vi "Autonomous Independent.vi"   [LabVIEW 2017] (continued)
                tunnel: w5039 -> [w5058]
                tunnel: w5038 -> [w5059]
                tunnel: [w5067] -> w5030
                tunnel: [w5066] -> w5031
                tunnel: [w5064] -> w5032
                tunnel: [w5065] -> w5033
                tunnel: w5037 -> [w5071]
                tunnel: w5036 -> [w5068]
                tunnel: w5035 -> [w5069]
                tunnel: w5034 -> [w5070]
                tunnel: [w5079] -> w5029
                tunnel: w5033 -> [w5075]
                tunnel: w5032 -> [w5076]
                tunnel: w5031 -> [w5078]
                tunnel: w5030 -> [w5080]
                tunnel: [w5077] -> w5028
                tunnel: [w5076] -> w5027
                tunnel: [w5075] -> w5026
                tunnel: w5029 -> [w5090]
                tunnel: [w5090] -> w5025
                tunnel: w5028 -> [w5089]
                tunnel: [w5089] -> w5024
                tunnel: [w5088] -> w5023
                tunnel: [w5087] -> w5022
                tunnel: w5027 -> [w5085]
                tunnel: w5026 -> [w5084]
                tunnel: w5025 -> [w5096]
                tunnel: [w5094] -> w5021
                tunnel: w5024 -> [w5095]
                tunnel: [w5093] -> w5020
                tunnel: w5023 -> [w5098]
                tunnel: w5022 -> [w5097]
                tunnel: [w5092] -> w5019
                tunnel: [w5091] -> w5018
                tunnel: w5021 -> [w5105]
                tunnel: [w5104] -> w5017
                tunnel: [w5103] -> w5016
                tunnel: w5020 -> [w5103]
                tunnel: [w5102] -> w5015
                tunnel: w5019 -> [w5102]
                tunnel: [w5101] -> w5014
                tunnel: w5018 -> [w5101]
                tunnel: [w5116] -> w5013
                tunnel: w5017 -> [w5116]
                tunnel: [w5115] -> w5012
                tunnel: w5016 -> [w5115]
                tunnel: [w5114] -> w5011
                tunnel: w5015 -> [w5114]
                tunnel: [w5113] -> w5010
                tunnel: w5014 -> [w5113]
                tunnel: w5013 -> [w5121]
                tunnel: w5012 -> [w5122]
                tunnel: [w5122] -> w5009
                tunnel: [w5121] -> w5008
                tunnel: [w5120] -> w5007
                tunnel: w5011 -> [w5120]
                tunnel: [w5119] -> w5006
                tunnel: w5010 -> [w5119]
                tunnel: [w5135] -> w5005
                tunnel: w5009 -> [w5137]
                tunnel: w5008 -> [w5136]
                tunnel: w5007 -> [w5132]
                tunnel: w5006 -> [w5131]
                tunnel: [w5130] -> w5004
                tunnel: [w5129] -> w5003
                tunnel: [w5128] -> w5002
                tunnel: w4997 -> [_]
                tunnel: w5005 -> [_]
                tunnel: w5004 -> [_]
                tunnel: w5003 -> [_]
                tunnel: w5002 -> [_]
                frame #0 {
                  n1471 = call "PID Distance.vi"("Distance"=20.0, "Angle"=2.0, "RightEncoder"=w5042, "LeftEncoder"=w5043, "GyroDevRef"=w5044, "RobotDriveDevRef"=w5045) -> ("RightEncoder 2"=w5046:T11, "LeftEncoder 2"=w5047:T11, "GyroDevRef 2"=w5048:T8, "RobotDriveDevRef 2"=w5049:T1)  [unwired: 2 in]
                }
                frame #1 {
                  n1472 = call "PID Distance.vi"("Distance"=100.0, "Angle"=2.0, "RightEncoder"=w5057, "LeftEncoder"=w5058, "GyroDevRef"=w5059, "RobotDriveDevRef"=w5060) -> ("RightEncoder 2"=w5053:T11, "LeftEncoder 2"=w5054:T11, "GyroDevRef 2"=w5055:T8, "RobotDriveDevRef 2"=w5056:T1)  [unwired: 2 in]
                  n1473 = global write "Robot Global Data.vi" "Raise_Mast"(TRUE ("Current State")) -> ()
                }
                frame #2 {
                  n1474 = global write "Robot Global Data.vi" "Lift_Position"(2.0) -> ()
                  n1475 = call "PID Distance.vi"("Distance"=300.0, "Angle"=2.0, "RightEncoder"=w5068, "LeftEncoder"=w5069, "GyroDevRef"=w5070, "RobotDriveDevRef"=w5071) -> ("RightEncoder 2"=w5064:T11, "LeftEncoder 2"=w5065:T11, "GyroDevRef 2"=w5066:T8, "RobotDriveDevRef 2"=w5067:T1)  [unwired: 2 in]
                  n1476 = global write "Robot Global Data.vi" "Raise_Mast"(TRUE ("Current State")) -> ()
                }
                frame #3 {
                  n1477 = global write "Robot Global Data.vi" "Lift_Position"(3.0) -> ()
                  n1478 = call "PID turning.vi"("Angle"=-90.0, "GyroDevRef"=w5078, "RobotDriveDevRef"=w5080) -> ("GyroDevRef 2"=w5077:T8, "RobotDriveDevRef 2"=w5079:T1)  [unwired: 7 in]
                  n1479 = global write "Robot Global Data.vi" "Raise_Mast"(TRUE ("Current State")) -> ()
                }
                frame #4 {
                  n1480 = call <vilib>:"WPI_EncoderReset.vi"("EncoderDevRef"=w5084) -> ("EncoderDevRef"=w5087:T11)  [unwired: 9 in, 1 out]
                  n1481 = Wait (ms)(milliseconds to wait=u32 10) -> ()  [unwired: 1 out]
                  n1482 = call <vilib>:"WPI_EncoderReset.vi"("EncoderDevRef"=w5085) -> ("EncoderDevRef"=w5088:T11)  [unwired: 9 in, 1 out]
                }
                frame #5 {
                  n1483 = call "PID Distance.vi"("Distance"=25.0, "Angle"=-90.0, "RightEncoder"=w5098, "LeftEncoder"=w5097, "GyroDevRef"=w5095, "RobotDriveDevRef"=w5096) -> ("RightEncoder 2"=w5091:T11, "LeftEncoder 2"=w5092:T11, "GyroDevRef 2"=w5093:T8, "RobotDriveDevRef 2"=w5094:T1)  [unwired: 2 in]
                }
                frame #6 {
                  w5106 = 0.0 ("Left axis value")
                  n1484 = global read "Robot Global Data.vi" "Axes"() -> (w5109:dbl[])
                  n1485 = Wait (ms)(milliseconds to wait=u32 500) -> ()  [unwired: 1 out]
                  n1486 = Array To Cluster(array=w5109) -> (cluster=w5108:T15)
                  n1487 = Bundle By Name(cluster=w5108, "Axes[1]"=0.25) -> (w5111:T15)
                  n1488 = Cluster To Array(cluster=w5111) -> (array=w5110:dbl[])
                  n1489 = call <vilib>:"WPI_RobotDriveTankDrive.vi"("Right axis value"=w5106, "Left axis value"=w5106, "RobotDriveDevRef"=w5105) -> ("RobotDriveDevRef"=w5104:T1)  [unwired: 6 in, 2 out]
                  n1490 = global write "Robot Global Data.vi" "Axes"(w5110) -> ()
                }
                frame #7 {
                  n1491 = global write "Robot Global Data.vi" "Current State"(FALSE ("Current State")) -> ()
                  n1492 = Wait (ms)(milliseconds to wait=u32 400) -> ()  [unwired: 1 out]
                }
                frame #8 {
                  n1493 = global read "Robot Global Data.vi" "Axes"() -> (w5124:dbl[])
                  n1494 = Array To Cluster(array=w5124) -> (cluster=w5123:T15)
                  n1495 = Bundle By Name(cluster=w5123, "Axes[1]"=-1.0) -> (w5126:T15)
                  n1496 = Cluster To Array(cluster=w5126) -> (array=w5125:dbl[])
                  n1497 = global write "Robot Global Data.vi" "Axes"(w5125) -> ()
                }
                frame #9 {
                  n1498 = call "PID Distance.vi"("Distance"=0.0, "Angle"=-90.0, "RightEncoder"=w5131, "LeftEncoder"=w5132, "GyroDevRef"=w5137, "RobotDriveDevRef"=w5136) -> ("RightEncoder 2"=w5128:T11, "LeftEncoder 2"=w5129:T11, "GyroDevRef 2"=w5130:T8, "RobotDriveDevRef 2"=w5135:T1)  [unwired: 2 in]
                }
                frame #10 {
                  n1499 = global write "Robot Global Data.vi" "Lift_Position"(1.0) -> ()
                }
              }
            }
            frame Default {
              n1500 = flat-sequence {
                tunnel: w5142 -> [w5148]
                tunnel: w5141 -> [w5147]
                tunnel: w5140 -> [w5145]
                tunnel: [w5146] -> w5143
                tunnel: w5139 -> [w5144]
                tunnel: w5143 -> [w5151]
                frame #0 {
                  n1501 = call "PID Distance.vi"("Distance"=90.0, "Angle"=0.0, "RightEncoder"=w5144, "LeftEncoder"=w5145, "GyroDevRef"=w5147, "RobotDriveDevRef"=w5148) -> ("RobotDriveDevRef 2"=w5146:T1)  [unwired: 2 in, 3 out]
                }
                frame #1 {
                  w5152 = 0.0
                  n1502 = call <vilib>:"WPI_RobotDriveTankDrive.vi"("Right axis value"=w5152, "Left axis value"=w5152, "RobotDriveDevRef"=w5151) -> ()  [unwired: 6 in, 3 out]
                }
              }
            }
          }
        }
      }
    }
    frame "Right Scale 2" {
      n1503 = flat-sequence {
        tunnel: w5158 -> [w5188]
        tunnel: w5155 -> [w5186]
        tunnel: w5156 -> [w5185]
        tunnel: w5157 -> [w5184]
        tunnel: [w5183] -> w5163
        tunnel: [w5182] -> w5162
        tunnel: [w5181] -> w5161
        tunnel: [w5180] -> w5160
        tunnel: w5159 -> [w5173]
        tunnel: w5154 -> [w5190]
        tunnel: w5163 -> [w5194]
        tunnel: w5162 -> [w5193]
        tunnel: w5161 -> [w5192]
        tunnel: w5160 -> [w5191]
        tunnel: w5153 -> [w5189]
        frame #0 {
          w5187 = 0.0 ("Left axis value")
          n1504 = global read "Robot Global Data.vi" "Axes"() -> (w5166:dbl[])
          n1505 = Multiply(x=w5173, y=1000.0) -> (x*y=w5174:dbl)
          n1506 = global write "Robot Global Data.vi" "Lift_Position"(0.0) -> ()
          n1507 = global write "Robot Global Data.vi" "Current State"(TRUE ("Current State")) -> ()
          n1508 = global write "Robot Global Data.vi" "Raise_Mast"(FALSE ("Current State")) -> ()
          n1509 = Wait (ms)(milliseconds to wait=u32 100) -> ()  [unwired: 1 out]
          n1510 = Array To Cluster(array=w5166) -> (cluster=w5165:T15)
          n1511 = Bundle By Name(cluster=w5165, "Axes[1]"=-1.0) -> (w5168:T15)
          n1512 = Greater?(x=w5174, y=11000.0) -> (0:w5176:bool)
          n1513 = Equal?(x=w5174, y=0.0) -> (x = y?=w5177:bool)
          n1514 = Or(x=w5176, y=w5177) -> ()  [unwired: 1 out]
          n1515 = Cluster To Array(cluster=w5168) -> (array=w5167:dbl[])
          n1516 = call <vilib>:"WPI_GyroReset.vi"("GyroDevRef"=w5184) -> ("GyroDevRef"=w5180:T8)  [unwired: 9 in, 1 out]
          n1517 = call <vilib>:"WPI_EncoderReset.vi"("EncoderDevRef"=w5186) -> ("EncoderDevRef"=w5182:T11)  [unwired: 9 in, 1 out]
          n1518 = global write "Robot Global Data.vi" "Axes"(w5167) -> ()
          n1519 = call <vilib>:"WPI_EncoderReset.vi"("EncoderDevRef"=w5185) -> ("EncoderDevRef"=w5181:T11)  [unwired: 9 in, 1 out]
          n1520 = call <vilib>:"WPI_RobotDriveTankDrive.vi"("Right axis value"=w5187, "Left axis value"=w5187, "RobotDriveDevRef"=w5188) -> ("RobotDriveDevRef"=w5183:T1)  [unwired: 6 in, 2 out]
        }
        frame #1 {
          n1521 = case shown="\"L\"" w5190 {
            tunnel: w5194 -> [w5196 w5543 w5871]
            tunnel: w5193 -> [w5199 w5540 w5873]
            tunnel: w5192 -> [w5198 w5541 w5872]
            tunnel: w5191 -> [w5197 w5542 w5870]
            tunnel: w5189 -> [w5195 w5539 _]
            frame "L" {
              n1522 = flat-sequence {
                tunnel: w5199 -> [w5261]
                tunnel: w5198 -> [w5262]
                tunnel: w5197 -> [w5263]
                tunnel: w5196 -> [w5264]
                tunnel: [w5257] -> w5255
                tunnel: [w5258] -> w5254
                tunnel: [w5259] -> w5253
                tunnel: [w5260] -> w5252
                tunnel: [w5274] -> w5251
                tunnel: [w5273] -> w5250
                tunnel: [w5271] -> w5249
                tunnel: [w5272] -> w5248
                tunnel: w5255 -> [w5270]
                tunnel: w5254 -> [w5269]
                tunnel: w5253 -> [w5268]
                tunnel: w5252 -> [w5267]
                tunnel: w5251 -> [w5280]
                tunnel: w5250 -> [w5281]
                tunnel: [w5284] -> w5247
                tunnel: w5249 -> [w5284]
                tunnel: [w5283] -> w5246
                tunnel: w5248 -> [w5283]
                tunnel: [w5278] -> w5245
                tunnel: [w5279] -> w5244
                tunnel: w5247 -> [w5291]
                tunnel: w5246 -> [w5290]
                tunnel: [w5289] -> w5243
                tunnel: [w5288] -> w5242
                tunnel: [w5287] -> w5241
                tunnel: w5245 -> [w5287]
                tunnel: [w5285] -> w5240
                tunnel: w5244 -> [w5285]
                tunnel: w5243 -> [w5296]
                tunnel: w5242 -> [w5297]
                tunnel: w5241 -> [w5298]
                tunnel: [w5294] -> w5239
                tunnel: [w5295] -> w5238
                tunnel: w5240 -> [w5299]
                tunnel: [w5292] -> w5237
                tunnel: [w5293] -> w5236
                tunnel: w5239 -> [w5311]
                tunnel: w5238 -> [w5310]
                tunnel: [w5309] -> w5235
                tunnel: [w5308] -> w5234
                tunnel: [w5314] -> w5233
                tunnel: w5237 -> [w5314]
                tunnel: [w5313] -> w5232
                tunnel: w5236 -> [w5313]
                tunnel: w5235 -> [w5320]
                tunnel: [w5320] -> w5231
                tunnel: [w5319] -> w5230
                tunnel: [w5318] -> w5229
                tunnel: [w5317] -> w5228
                tunnel: w5234 -> [w5317]
                tunnel: w5233 -> [w5316]
                tunnel: w5232 -> [w5315]
                tunnel: w5231 -> [w5328]
                tunnel: [w5325] -> w5227
                tunnel: w5230 -> [w5327]
                tunnel: w5229 -> [w5326]
                tunnel: w5228 -> [w5329]
                tunnel: [w5324] -> w5226
                tunnel: [w5323] -> w5225
                tunnel: [w5322] -> w5224
                tunnel: w5227 -> [w5336]
                tunnel: [w5335] -> w5223
                tunnel: w5226 -> [w5333]
                tunnel: [w5332] -> w5222
                tunnel: w5225 -> [w5338]
                tunnel: [w5338] -> w5221
                tunnel: w5224 -> [w5337]
                tunnel: [w5337] -> w5220
                tunnel: w5223 -> [w5349]
                tunnel: [w5343] -> w5219
                tunnel: [w5342] -> w5218
                tunnel: w5222 -> [w5342]
                tunnel: [w5341] -> w5217
                tunnel: w5221 -> [w5341]
                tunnel: [w5340] -> w5216
                tunnel: w5220 -> [w5340]
                tunnel: w5219 -> [w5356]
                tunnel: [w5356] -> w5215
                tunnel: w5218 -> [w5355]
                tunnel: [w5355] -> w5214
                tunnel: w5217 -> [w5354]
                tunnel: [w5354] -> w5213
                tunnel: w5216 -> [w5353]
                tunnel: [w5353] -> w5212
                tunnel: w5215 -> [w5360]
                tunnel: [w5358] -> w5211
                tunnel: w5214 -> [w5359]
                tunnel: [w5357] -> w5210
                tunnel: w5213 -> [w5363]
                tunnel: [w5363] -> w5209
                tunnel: w5212 -> [w5362]
                tunnel: [w5362] -> w5208
                tunnel: w5211 -> [w5376]
                tunnel: w5210 -> [w5375]
                tunnel: w5209 -> [w5374]
                tunnel: w5208 -> [w5373]
                tunnel: [w5367] -> w5207
                tunnel: [w5366] -> w5206
                tunnel: [w5365] -> w5205
                tunnel: [w5364] -> w5204
                tunnel: w5207 -> [w5383]
                tunnel: [w5383] -> w5203
                tunnel: w5206 -> [w5382]
                tunnel: [w5382] -> w5202
                tunnel: w5205 -> [w5381]
                tunnel: [w5381] -> w5201
                tunnel: w5204 -> [w5380]
                tunnel: [w5380] -> w5200
                tunnel: w5203 -> [w5388]
                tunnel: w5202 -> [w5387]
                tunnel: w5201 -> [w5385]
                tunnel: w5200 -> [w5386]
                tunnel: w5195 -> [w5384]
                frame #0 {
                  n1523 = global write "Robot Global Data.vi" "Raise_Mast"(FALSE ("Current State")) -> ()
                  n1524 = call "PID Distance.vi"("Distance"=20.0, "Angle"=0.0, "RightEncoder"=w5261, "LeftEncoder"=w5262, "GyroDevRef"=w5263, "RobotDriveDevRef"=w5264) -> ("RightEncoder 2"=w5260:T11, "LeftEncoder 2"=w5259:T11, "GyroDevRef 2"=w5258:T8, "RobotDriveDevRef 2"=w5257:T1)  [unwired: 2 in]
                }
                frame #1 {
                  n1525 = global write "Robot Global Data.vi" "Raise_Mast"(TRUE ("Current State")) -> ()
                  n1526 = call "PID Distance.vi"("Distance"=225.0, "Angle"=0.0, "RightEncoder"=w5267, "LeftEncoder"=w5268, "GyroDevRef"=w5269, "RobotDriveDevRef"=w5270) -> ("RightEncoder 2"=w5271:T11, "LeftEncoder 2"=w5272:T11, "GyroDevRef 2"=w5273:T8, "RobotDriveDevRef 2"=w5274:T1)  [unwired: 2 in]
                }
                frame #2 {
                  n1527 = call "PID turning.vi"("Angle"=-90.0, "GyroDevRef"=w5281, "RobotDriveDevRef"=w5280) -> ("GyroDevRef 2"=w5278:T8, "RobotDriveDevRef 2"=w5279:T1)  [unwired: 7 in]
                }
                frame #3 {
                  n1528 = call <vilib>:"WPI_EncoderReset.vi"("EncoderDevRef"=w5290) -> ("EncoderDevRef"=w5288:T11)  [unwired: 9 in, 1 out]
                  n1529 = Wait (ms)(milliseconds to wait=u32 10) -> ()  [unwired: 1 out]
                  n1530 = call <vilib>:"WPI_EncoderReset.vi"("EncoderDevRef"=w5291) -> ("EncoderDevRef"=w5289:T11)  [unwired: 9 in, 1 out]
                }
                frame #4 {
                  n1531 = global read "Robot Global Data.vi" "Axes"() -> (w5303:dbl[])
                  n1532 = global write "Robot Global Data.vi" "Lift_Position"(2.0) -> ()
                  n1533 = call "PID Distance.vi"("Distance"=199.0, "Angle"=-90.0, "RightEncoder"=w5296, "LeftEncoder"=w5297, "GyroDevRef"=w5298, "RobotDriveDevRef"=w5299) -> ("RightEncoder 2"=w5293:T11, "LeftEncoder 2"=w5292:T11, "GyroDevRef 2"=w5295:T8, "RobotDriveDevRef 2"=w5294:T1)  [unwired: 2 in]
                  n1534 = Array To Cluster(array=w5303) -> (cluster=w5302:T15)
                  n1535 = Bundle By Name(cluster=w5302, "Axes[1]"=-1.0) -> (w5301:T15)
                  n1536 = Cluster To Array(cluster=w5301) -> (array=w5300:dbl[])
                  n1537 = global write "Robot Global Data.vi" "Axes"(w5300) -> ()
                }
                frame #5 {
                  n1538 = call "PID turning.vi"("Angle"=0.0, "GyroDevRef"=w5310, "RobotDriveDevRef"=w5311) -> ("GyroDevRef 2"=w5308:T8, "RobotDriveDevRef 2"=w5309:T1)  [unwired: 7 in]
                }
                frame #6 {
                  n1539 = call <vilib>:"WPI_EncoderReset.vi"("EncoderDevRef"=w5316) -> ("EncoderDevRef"=w5319:T11)  [unwired: 9 in, 1 out]
                  n1540 = call <vilib>:"WPI_EncoderReset.vi"("EncoderDevRef"=w5315) -> ("EncoderDevRef"=w5318:T11)  [unwired: 9 in, 1 out]
                }
                frame #7 {
                  n1541 = call "PID Distance.vi"("Distance"=38.0, "Angle"=0.0, "RightEncoder"=w5326, "LeftEncoder"=w5327, "GyroDevRef"=w5329, "RobotDriveDevRef"=w5328) -> ("RightEncoder 2"=w5322:T11, "LeftEncoder 2"=w5323:T11, "GyroDevRef 2"=w5324:T8, "RobotDriveDevRef 2"=w5325:T1)  [unwired: 2 in]
                  n1542 = global write "Robot Global Data.vi" "Lift_Position"(3.0) -> ()
                }
                frame #8 {
                  n1543 = call "PID turning.vi"("Angle"=20.0, "GyroDevRef"=w5333, "RobotDriveDevRef"=w5336) -> ("GyroDevRef 2"=w5332:T8, "RobotDriveDevRef 2"=w5335:T1)  [unwired: 7 in]
                }
                frame #9 {
                  w5350 = 0.0 ("Left axis value")
                  n1544 = global read "Robot Global Data.vi" "Axes"() -> (w5345:dbl[])
                  n1545 = Wait (ms)(milliseconds to wait=u32 300) -> ()  [unwired: 1 out]
                  n1546 = Array To Cluster(array=w5345) -> (cluster=w5344:T15)
                  n1547 = Bundle By Name(cluster=w5344, "Axes[1]"=0.25) -> (w5347:T15)
                  n1548 = Cluster To Array(cluster=w5347) -> (array=w5346:dbl[])
                  n1549 = call <vilib>:"WPI_RobotDriveTankDrive.vi"("Right axis value"=w5350, "Left axis value"=w5350, "RobotDriveDevRef"=w5349) -> ("RobotDriveDevRef"=w5343:T1)  [unwired: 6 in, 2 out]
                  n1550 = global write "Robot Global Data.vi" "Axes"(w5346) -> ()
                }
                frame #10 {
                  n1551 = global write "Robot Global Data.vi" "Current State"(FALSE ("Current State")) -> ()
                  n1552 = Wait (ms)(milliseconds to wait=u32 400) -> ()  [unwired: 1 out]
                }
                frame #11 {
                  n1553 = call "PID turning.vi"("Angle"=0.0, "GyroDevRef"=w5359, "RobotDriveDevRef"=w5360) -> ("GyroDevRef 2"=w5357:T8, "RobotDriveDevRef 2"=w5358:T1)  [unwired: 7 in]
                }
                frame #12 {
                  n1554 = global read "Robot Global Data.vi" "Axes"() -> (w5372:dbl[])
                  n1555 = Array To Cluster(array=w5372) -> (cluster=w5371:T15)
                  n1556 = call "PID Distance.vi"("Distance"=0.0, "Angle"=0.0, "RightEncoder"=w5373, "LeftEncoder"=w5374, "GyroDevRef"=w5375, "RobotDriveDevRef"=w5376) -> ("RightEncoder 2"=w5364:T11, "LeftEncoder 2"=w5365:T11, "GyroDevRef 2"=w5366:T8, "RobotDriveDevRef 2"=w5367:T1)  [unwired: 2 in]
                  n1557 = Bundle By Name(cluster=w5371, "Axes[1]"=-1.0) -> (w5370:T15)
                  n1558 = Cluster To Array(cluster=w5370) -> (array=w5369:dbl[])
                  n1559 = global write "Robot Global Data.vi" "Axes"(w5369) -> ()
                }
                frame #13 {
                  n1560 = global write "Robot Global Data.vi" "Lift_Position"(1.0) -> ()
                }
                frame #14 {
                  n1561 = case shown="\"L\"" w5384 {
                    tunnel: w5388 -> [w5392 w5463 _]
                    tunnel: w5387 -> [w5391 w5462 _]
                    tunnel: w5386 -> [w5390 w5459 _]
                    tunnel: w5385 -> [w5389 w5458 _]
                    frame "R" {
                      n1562 = flat-sequence {
                        tunnel: w5392 -> [w5401]
                        tunnel: w5391 -> [w5400]
                        tunnel: [w5403] -> w5398
                        tunnel: [w5402] -> w5397
                        tunnel: w5398 -> [w5410]
                        tunnel: w5397 -> [w5409]
                        tunnel: [w5410] -> w5393
                        tunnel: [w5409] -> w5394
                        tunnel: [w5407] -> w5395
                        tunnel: [w5406] -> w5396
                        tunnel: w5390 -> [w5405]
                        tunnel: w5389 -> [w5404]
                        tunnel: w5396 -> [w5412]
                        tunnel: w5395 -> [w5413]
                        tunnel: w5394 -> [w5414]
                        tunnel: w5393 -> [w5415]
                        frame #0 {
                          n1563 = call "PID turning.vi"("Angle"=170.0, "GyroDevRef"=w5400, "RobotDriveDevRef"=w5401) -> ("GyroDevRef 2"=w5402:T8, "RobotDriveDevRef 2"=w5403:T1)  [unwired: 7 in]
                        }
                        frame #1 {
                          n1564 = call <vilib>:"WPI_EncoderReset.vi"("EncoderDevRef"=w5405) -> ("EncoderDevRef"=w5406:T11)  [unwired: 9 in, 1 out]
                          n1565 = Wait (ms)(milliseconds to wait=u32 10) -> ()  [unwired: 1 out]
                          n1566 = call <vilib>:"WPI_EncoderReset.vi"("EncoderDevRef"=w5404) -> ("EncoderDevRef"=w5407:T11)  [unwired: 9 in, 1 out]
                        }
                        frame #2 {
                          n1567 = global read "Robot Global Data.vi" "Axes"() -> (w5421:dbl[])
                          n1568 = Wait (ms)(milliseconds to wait=u32 400) -> ()  [unwired: 1 out]
                          n1569 = Array To Cluster(array=w5421) -> (cluster=w5422:T15)
                          n1570 = Bundle By Name(cluster=w5422, "Axes[1]"=1.0) -> (w5423:T15)
                          n1571 = global read "Robot Global Data.vi" "PIXY Output"() -> (w5411:T16)
                          n1572 = Unbundle By Name(w5411) -> ("SIGNATURE NUMBER"=w5418:u16)
                          n1573 = global read "Robot Global Data.vi" "Cube Signature"() -> (w5416:dbl)
                          n1574 = Equal?(x=w5418, y=w5416) -> (x = y?=w5417:bool)
                          n1575 = Cluster To Array(cluster=w5423) -> (array=w5424:dbl[])
                          n1576 = global write "Robot Global Data.vi" "Axes"(w5424) -> ()
                          n1577 = case shown="False" w5417 {
                            tunnel: [w5426 w5439] -> _
                            tunnel: [w5425 w5438] -> _
                            tunnel: [w5428 w5437] -> _
                            tunnel: [w5429 w5436] -> _
                            tunnel: w5415 -> [w5427 w5433]
                            tunnel: w5414 -> [w5428 w5432]
                            tunnel: w5413 -> [w5425 w5431]
                            tunnel: w5412 -> [w5426 w5430]
                            frame True {
                              n1578 = call "PID vision.vi"("RobotDriveDevRef in"=w5427) -> ("RobotDriveDevRef out"=w5429:T1)  [unwired: 9 in, 1 out]
                            }
                            frame False {
                              n1579 = call "PID Distance.vi"("Distance"=45.0, "Angle"=170.0, "RightEncoder"=w5430, "LeftEncoder"=w5431, "GyroDevRef"=w5432, "RobotDriveDevRef"=w5433) -> ("RightEncoder 2"=w5439:T11, "LeftEncoder 2"=w5438:T11, "GyroDevRef 2"=w5437:T8, "RobotDriveDevRef 2"=w5436:T1)  [unwired: 2 in]
                            }
                          }
                        }
                        frame #3 {
                          n1580 = global write "Robot Global Data.vi" "Current State"(TRUE ("Current State")) -> ()
                          n1581 = Wait (ms)(milliseconds to wait=u32 300) -> ()  [unwired: 1 out]
                        }
                      }
                    }
                    frame "L" {
                      n1582 = flat-sequence {
                        tunnel: w5463 -> [w5466]
                        tunnel: w5462 -> [w5465]
                        tunnel: [w5468] -> w5461
                        tunnel: [w5467] -> w5460
                        tunnel: w5461 -> [w5475]
                        tunnel: w5460 -> [w5474]
                        tunnel: w5459 -> [w5472]
                        tunnel: w5458 -> [w5471]
                        tunnel: [w5475] -> w5457
                        tunnel: [w5474] -> w5456
                        tunnel: [w5470] -> w5455
                        tunnel: [w5469] -> w5454
                        tunnel: [w5493] -> w5453
                        tunnel: [w5492] -> w5452
                        tunnel: [w5491] -> w5451
                        tunnel: [w5490] -> w5450
                        tunnel: w5454 -> [w5482]
                        tunnel: w5455 -> [w5483]
                        tunnel: w5456 -> [w5481]
                        tunnel: w5457 -> [w5480]
                        tunnel: w5453 -> [w5514]
                        tunnel: w5452 -> [w5513]
                        tunnel: w5451 -> [w5512]
                        tunnel: w5450 -> [w5511]
                        tunnel: [w5514] -> w5449
                        tunnel: [w5513] -> w5447
                        tunnel: [w5512] -> w5445
                        tunnel: [w5511] -> w5443
                        tunnel: w5449 -> [w5525]
                        tunnel: [w5525] -> w5448
                        tunnel: w5447 -> [w5524]
                        tunnel: [w5524] -> w5446
                        tunnel: w5445 -> [w5523]
                        tunnel: [w5523] -> w5444
                        tunnel: w5443 -> [w5522]
                        tunnel: [w5522] -> w5442
                        tunnel: w5448 -> [w5526]
                        tunnel: w5446 -> [w5529]
                        tunnel: w5444 -> [w5528]
                        tunnel: w5442 -> [w5527]
                        frame #0 {
                          n1583 = call "PID turning.vi"("Angle"=170.0, "GyroDevRef"=w5465, "RobotDriveDevRef"=w5466) -> ("GyroDevRef 2"=w5467:T8, "RobotDriveDevRef 2"=w5468:T1)  [unwired: 7 in]
                        }
                        frame #1 {
                          n1584 = call <vilib>:"WPI_EncoderReset.vi"("EncoderDevRef"=w5471) -> ("EncoderDevRef"=w5469:T11)  [unwired: 9 in, 1 out]
                          n1585 = Wait (ms)(milliseconds to wait=u32 10) -> ()  [unwired: 1 out]
                          n1586 = call <vilib>:"WPI_EncoderReset.vi"("EncoderDevRef"=w5472) -> ("EncoderDevRef"=w5470:T11)  [unwired: 9 in, 1 out]
                        }
                        frame #2 {
                          n1587 = global read "Robot Global Data.vi" "Axes"() -> (w5486:dbl[])
                          n1588 = Wait (ms)(milliseconds to wait=u32 400) -> ()  [unwired: 1 out]
                          n1589 = Array To Cluster(array=w5486) -> (cluster=w5487:T15)
                          n1590 = Bundle By Name(cluster=w5487, "Axes[1]"=1.0) -> (w5488:T15)
                          n1591 = global read "Robot Global Data.vi" "PIXY Output"() -> (w5476:T16)
                          n1592 = Unbundle By Name(w5476) -> ("SIGNATURE NUMBER"=w5479:u16)
                          n1593 = global read "Robot Global Data.vi" "Cube Signature"() -> (w5477:dbl)
                          n1594 = Equal?(x=w5479, y=w5477) -> (x = y?=w5478:bool)
                          n1595 = Cluster To Array(cluster=w5488) -> (array=w5489:dbl[])
                          n1596 = global write "Robot Global Data.vi" "Axes"(w5489) -> ()
                          n1597 = case shown="True" w5478 {
                            tunnel: [w5495 w5508] -> w5493
                            tunnel: [w5494 w5507] -> w5492
                            tunnel: [w5496 w5506] -> w5491
                            tunnel: [w5497 w5505] -> w5490
                            tunnel: w5483 -> [w5494 w5502]
                            tunnel: w5482 -> [w5495 w5501]
                            tunnel: w5481 -> [w5496 w5500]
                            tunnel: w5480 -> [w5498 w5499]
                            frame True {
                              (unwired) 10.0 ("Distance")
                              n1598 = call "PID vision.vi"("RobotDriveDevRef in"=w5498) -> ("RobotDriveDevRef out"=w5497:T1)  [unwired: 9 in, 1 out]
                            }
                            frame False {
                              n1599 = call "PID Distance.vi"("Distance"=45.0, "Angle"=170.0, "RightEncoder"=w5502, "LeftEncoder"=w5501, "GyroDevRef"=w5500, "RobotDriveDevRef"=w5499) -> ("RightEncoder 2"=w5508:T11, "LeftEncoder 2"=w5507:T11, "GyroDevRef 2"=w5506:T8, "RobotDriveDevRef 2"=w5505:T1)  [unwired: 2 in]
                            }
                          }
                        }
                        frame #3 {
                          n1600 = global write "Robot Global Data.vi" "Current State"(TRUE ("Current State")) -> ()
                          n1601 = Wait (ms)(milliseconds to wait=u32 500) -> ()  [unwired: 1 out]
                        }
                        frame #4 {
                          n1602 = global read "Robot Global Data.vi" "Axes"() -> (w5520:dbl[])
                          n1603 = global write "Robot Global Data.vi" "Lift_Position"(2.0) -> ()
                          n1604 = Wait (ms)(milliseconds to wait=u32 250) -> ()  [unwired: 1 out]
                          n1605 = Array To Cluster(array=w5520) -> (cluster=w5519:T15)
                          n1606 = Bundle By Name(cluster=w5519, "Axes[1]"=-1.0) -> (w5517:T15)
                          n1607 = Cluster To Array(cluster=w5517) -> (array=w5516:dbl[])
                          n1608 = global write "Robot Global Data.vi" "Axes"(w5516) -> ()
                        }
                        frame #5 {
                          n1609 = call "PID Distance.vi"("Distance"=60.0, "Angle"=170.0, "RightEncoder"=w5526, "LeftEncoder"=w5529, "GyroDevRef"=w5528, "RobotDriveDevRef"=w5527) -> ()  [unwired: 2 in, 4 out]
                        }
                        frame #6 {
                          n1610 = global read "Robot Global Data.vi" "Axes"() -> (w5537:dbl[])
                          n1611 = Wait (ms)(milliseconds to wait=u32 250) -> ()  [unwired: 1 out]
                          n1612 = Array To Cluster(array=w5537) -> (cluster=w5536:T15)
                          n1613 = Bundle By Name(cluster=w5536, "Axes[1]"=1.0) -> (w5534:T15)
                          n1614 = Cluster To Array(cluster=w5534) -> (array=w5533:dbl[])
                          n1615 = global write "Robot Global Data.vi" "Axes"(w5533) -> ()
                        }
                        frame #7 {
                          n1616 = global write "Robot Global Data.vi" "Current State"(FALSE ("Current State")) -> ()
                        }
                      }
                    }
                    frame Default {
                    }
                  }
                }
              }
            }
            frame "R" {
              n1617 = flat-sequence {
                tunnel: [w5607] -> w5599
                tunnel: [w5604] -> w5598
                tunnel: [w5605] -> w5597
                tunnel: [w5606] -> w5596
                tunnel: w5543 -> [w5603]
                tunnel: w5542 -> [w5602]
                tunnel: w5541 -> [w5601]
                tunnel: w5540 -> [w5600]
                tunnel: [w5614] -> w5595
                tunnel: [w5611] -> w5594
                tunnel: [w5612] -> w5593
                tunnel: [w5613] -> w5592
                tunnel: w5599 -> [w5618]
                tunnel: w5598 -> [w5615]
                tunnel: w5597 -> [w5616]
                tunnel: w5596 -> [w5617]
                tunnel: [w5625] -> w5588
                tunnel: [w5624] -> w5589
                tunnel: [w5622] -> w5590
                tunnel: [w5623] -> w5591
                tunnel: w5595 -> [w5629]
                tunnel: w5594 -> [w5626]
                tunnel: w5593 -> [w5627]
                tunnel: w5592 -> [w5628]
                tunnel: [w5637] -> w5587
                tunnel: w5591 -> [w5633]
                tunnel: w5590 -> [w5634]
                tunnel: w5589 -> [w5636]
                tunnel: w5588 -> [w5638]
                tunnel: [w5635] -> w5586
                tunnel: [w5634] -> w5585
                tunnel: [w5633] -> w5584
                tunnel: w5587 -> [w5648]
                tunnel: [w5648] -> w5583
                tunnel: w5586 -> [w5647]
                tunnel: [w5647] -> w5582
                tunnel: [w5646] -> w5581
                tunnel: [w5645] -> w5580
                tunnel: w5585 -> [w5643]
                tunnel: w5584 -> [w5642]
                tunnel: w5583 -> [w5654]
                tunnel: [w5652] -> w5579
                tunnel: w5582 -> [w5653]
                tunnel: [w5651] -> w5578
                tunnel: w5581 -> [w5656]
                tunnel: w5580 -> [w5655]
                tunnel: [w5650] -> w5577
                tunnel: [w5649] -> w5576
                tunnel: w5579 -> [w5663]
                tunnel: [w5662] -> w5575
                tunnel: [w5661] -> w5574
                tunnel: w5578 -> [w5661]
                tunnel: [w5660] -> w5573
                tunnel: w5577 -> [w5660]
                tunnel: [w5659] -> w5572
                tunnel: w5576 -> [w5659]
                tunnel: [w5674] -> w5571
                tunnel: w5575 -> [w5674]
                tunnel: [w5673] -> w5570
                tunnel: w5574 -> [w5673]
                tunnel: [w5672] -> w5569
                tunnel: w5573 -> [w5672]
                tunnel: [w5671] -> w5568
                tunnel: w5572 -> [w5671]
                tunnel: w5571 -> [w5679]
                tunnel: w5570 -> [w5680]
                tunnel: [w5680] -> w5567
                tunnel: [w5679] -> w5566
                tunnel: [w5678] -> w5565
                tunnel: w5569 -> [w5678]
                tunnel: [w5677] -> w5564
                tunnel: w5568 -> [w5677]
                tunnel: [w5693] -> w5563
                tunnel: w5567 -> [w5695]
                tunnel: w5566 -> [w5694]
                tunnel: w5565 -> [w5690]
                tunnel: w5564 -> [w5689]
                tunnel: [w5688] -> w5562
                tunnel: [w5687] -> w5561
                tunnel: [w5686] -> w5560
                tunnel: w5563 -> [w5702]
                tunnel: w5562 -> [w5701]
                tunnel: [w5700] -> w5559
                tunnel: w5561 -> [w5700]
                tunnel: [w5699] -> w5558
                tunnel: w5560 -> [w5699]
                tunnel: [w5698] -> w5557
                tunnel: [w5697] -> w5556
                tunnel: w5559 -> [w5710]
                tunnel: w5558 -> [w5709]
                tunnel: [w5707] -> w5555
                tunnel: w5557 -> [w5707]
                tunnel: [w5706] -> w5554
                tunnel: w5556 -> [w5706]
                tunnel: [w5705] -> w5553
                tunnel: [w5704] -> w5552
                tunnel: w5555 -> [w5723]
                tunnel: w5554 -> [w5722]
                tunnel: w5553 -> [w5721]
                tunnel: w5552 -> [w5720]
                tunnel: [w5719] -> w5551
                tunnel: [w5718] -> w5550
                tunnel: [w5717] -> w5549
                tunnel: [w5716] -> w5548
                tunnel: [w5729] -> w5547
                tunnel: [w5726] -> w5546
                tunnel: [w5728] -> w5545
                tunnel: [w5727] -> w5544
                tunnel: w5548 -> [w5726]
                tunnel: w5549 -> [w5727]
                tunnel: w5550 -> [w5728]
                tunnel: w5551 -> [w5729]
                tunnel: w5547 -> [w5736]
                tunnel: w5546 -> [w5735]
                tunnel: w5545 -> [w5734]
                tunnel: w5544 -> [w5733]
                tunnel: w5539 -> [w5732]
                frame #0 {
                  n1618 = call "PID Distance.vi"("Distance"=20.0, "Angle"=2.0, "RightEncoder"=w5600, "LeftEncoder"=w5601, "GyroDevRef"=w5602, "RobotDriveDevRef"=w5603) -> ("RightEncoder 2"=w5604:T11, "LeftEncoder 2"=w5605:T11, "GyroDevRef 2"=w5606:T8, "RobotDriveDevRef 2"=w5607:T1)  [unwired: 2 in]
                }
                frame #1 {
                  n1619 = call "PID Distance.vi"("Distance"=100.0, "Angle"=2.0, "RightEncoder"=w5615, "LeftEncoder"=w5616, "GyroDevRef"=w5617, "RobotDriveDevRef"=w5618) -> ("RightEncoder 2"=w5611:T11, "LeftEncoder 2"=w5612:T11, "GyroDevRef 2"=w5613:T8, "RobotDriveDevRef 2"=w5614:T1)  [unwired: 2 in]
                  n1620 = global write "Robot Global Data.vi" "Raise_Mast"(TRUE ("Current State")) -> ()
                }
                frame #2 {
                  n1621 = global write "Robot Global Data.vi" "Lift_Position"(2.0) -> ()
                  n1622 = call "PID Distance.vi"("Distance"=300.0, "Angle"=2.0, "RightEncoder"=w5626, "LeftEncoder"=w5627, "GyroDevRef"=w5628, "RobotDriveDevRef"=w5629) -> ("RightEncoder 2"=w5622:T11, "LeftEncoder 2"=w5623:T11, "GyroDevRef 2"=w5624:T8, "RobotDriveDevRef 2"=w5625:T1)  [unwired: 2 in]
                  n1623 = global write "Robot Global Data.vi" "Raise_Mast"(TRUE ("Current State")) -> ()
                }
                frame #3 {
                  n1624 = global write "Robot Global Data.vi" "Lift_Position"(3.0) -> ()
                  n1625 = call "PID turning.vi"("Angle"=-90.0, "GyroDevRef"=w5636, "RobotDriveDevRef"=w5638) -> ("GyroDevRef 2"=w5635:T8, "RobotDriveDevRef 2"=w5637:T1)  [unwired: 7 in]
                  n1626 = global write "Robot Global Data.vi" "Raise_Mast"(TRUE ("Current State")) -> ()
                }
                frame #4 {
                  n1627 = call <vilib>:"WPI_EncoderReset.vi"("EncoderDevRef"=w5642) -> ("EncoderDevRef"=w5645:T11)  [unwired: 9 in, 1 out]
                  n1628 = Wait (ms)(milliseconds to wait=u32 100) -> ()  [unwired: 1 out]
                  n1629 = call <vilib>:"WPI_EncoderReset.vi"("EncoderDevRef"=w5643) -> ("EncoderDevRef"=w5646:T11)  [unwired: 9 in, 1 out]
                }
                frame #5 {
                  n1630 = call "PID Distance.vi"("Distance"=25.0, "Angle"=-90.0, "RightEncoder"=w5656, "LeftEncoder"=w5655, "GyroDevRef"=w5653, "RobotDriveDevRef"=w5654) -> ("RightEncoder 2"=w5649:T11, "LeftEncoder 2"=w5650:T11, "GyroDevRef 2"=w5651:T8, "RobotDriveDevRef 2"=w5652:T1)  [unwired: 2 in]
                }
                frame #6 {
                  w5664 = 0.0 ("Left axis value")
                  n1631 = global read "Robot Global Data.vi" "Axes"() -> (w5667:dbl[])
                  n1632 = Wait (ms)(milliseconds to wait=u32 500) -> ()  [unwired: 1 out]
                  n1633 = Array To Cluster(array=w5667) -> (cluster=w5666:T15)
                  n1634 = Bundle By Name(cluster=w5666, "Axes[1]"=0.25) -> (w5669:T15)
                  n1635 = Cluster To Array(cluster=w5669) -> (array=w5668:dbl[])
                  n1636 = call <vilib>:"WPI_RobotDriveTankDrive.vi"("Right axis value"=w5664, "Left axis value"=w5664, "RobotDriveDevRef"=w5663) -> ("RobotDriveDevRef"=w5662:T1)  [unwired: 6 in, 2 out]
                  n1637 = global write "Robot Global Data.vi" "Axes"(w5668) -> ()
                }
                frame #7 {
                  n1638 = global write "Robot Global Data.vi" "Current State"(FALSE ("Current State")) -> ()
                  n1639 = Wait (ms)(milliseconds to wait=u32 400) -> ()  [unwired: 1 out]
                }
                frame #8 {
                  n1640 = global read "Robot Global Data.vi" "Axes"() -> (w5682:dbl[])
                  n1641 = Array To Cluster(array=w5682) -> (cluster=w5681:T15)
                  n1642 = Bundle By Name(cluster=w5681, "Axes[1]"=-1.0) -> (w5684:T15)
                  n1643 = Cluster To Array(cluster=w5684) -> (array=w5683:dbl[])
                  n1644 = global write "Robot Global Data.vi" "Axes"(w5683) -> ()
                }
                frame #9 {
                  n1645 = call "PID Distance.vi"("Distance"=0.0, "Angle"=-90.0, "RightEncoder"=w5689, "LeftEncoder"=w5690, "GyroDevRef"=w5695, "RobotDriveDevRef"=w5694) -> ("RightEncoder 2"=w5686:T11, "LeftEncoder 2"=w5687:T11, "GyroDevRef 2"=w5688:T8, "RobotDriveDevRef 2"=w5693:T1)  [unwired: 2 in]
                }
                frame #10 {
                  n1646 = global write "Robot Global Data.vi" "Lift_Position"(1.0) -> ()
                  n1647 = call "PID turning.vi"("Angle"=-150.0, "GyroDevRef"=w5701, "RobotDriveDevRef"=w5702) -> ("GyroDevRef 2"=w5697:T8, "RobotDriveDevRef 2"=w5698:T1)  [unwired: 7 in]
                }
                frame #11 {
                  n1648 = call <vilib>:"WPI_EncoderReset.vi"("EncoderDevRef"=w5710) -> ("EncoderDevRef"=w5705:T11)  [unwired: 9 in, 1 out]
                  n1649 = Wait (ms)(milliseconds to wait=u32 10) -> ()  [unwired: 1 out]
                  n1650 = call <vilib>:"WPI_EncoderReset.vi"("EncoderDevRef"=w5709) -> ("EncoderDevRef"=w5704:T11)  [unwired: 9 in, 1 out]
                }
                frame #12 {
                  n1651 = global read "Robot Global Data.vi" "Axes"() -> (w5713:dbl[])
                  n1652 = call "PID Distance.vi"("Distance"=130.0, "Angle"=-150.0, "RightEncoder"=w5720, "LeftEncoder"=w5721, "GyroDevRef"=w5722, "RobotDriveDevRef"=w5723) -> ("RightEncoder 2"=w5716:T11, "LeftEncoder 2"=w5717:T11, "GyroDevRef 2"=w5718:T8, "RobotDriveDevRef 2"=w5719:T1)  [unwired: 2 in]
                  n1653 = Array To Cluster(array=w5713) -> (cluster=w5712:T15)
                  n1654 = Bundle By Name(cluster=w5712, "Axes[1]"=1.0) -> (w5715:T15)
                  n1655 = Cluster To Array(cluster=w5715) -> (array=w5714:dbl[])
                  n1656 = global write "Robot Global Data.vi" "Axes"(w5714) -> ()
                }
                frame #13 {
                  n1657 = global write "Robot Global Data.vi" "Current State"(TRUE ("Current State")) -> ()
                  n1658 = Wait (ms)(milliseconds to wait=u32 500) -> ()  [unwired: 1 out]
                }
                frame #14 {
                  n1659 = case shown="\"R\"" w5732 {
                    tunnel: w5736 -> [w5740 w5793 _]
                    tunnel: w5735 -> [w5739 w5792 _]
                    tunnel: w5734 -> [w5738 w5791 _]
                    tunnel: w5733 -> [w5737 w5790 _]
                    frame "R" {
                      n1660 = flat-sequence {
                        tunnel: w5740 -> [w5750]
                        tunnel: w5739 -> [w5751]
                        tunnel: w5738 -> [w5749]
                        tunnel: w5737 -> [w5748]
                        frame #0 {
                          n1661 = global read "Robot Global Data.vi" "Axes"() -> (w5745:dbl[])
                          n1662 = global write "Robot Global Data.vi" "Lift_Position"(2.0) -> ()
                          n1663 = Wait (ms)(milliseconds to wait=u32 250) -> ()  [unwired: 1 out]
                          n1664 = Array To Cluster(array=w5745) -> (cluster=w5744:T15)
                          n1665 = Bundle By Name(cluster=w5744, "Axes[1]"=-1.0) -> (w5747:T15)
                          n1666 = Cluster To Array(cluster=w5747) -> (array=w5746:dbl[])
                          n1667 = global write "Robot Global Data.vi" "Axes"(w5746) -> ()
                        }
                        frame #1 {
                          n1668 = call "PID Distance.vi"("Distance"=150.0, "Angle"=-170.0, "RightEncoder"=w5751, "LeftEncoder"=w5748, "GyroDevRef"=w5749, "RobotDriveDevRef"=w5750) -> ()  [unwired: 2 in, 4 out]
                        }
                        frame #2 {
                          n1669 = global read "Robot Global Data.vi" "Axes"() -> (w5757:dbl[])
                          n1670 = Wait (ms)(milliseconds to wait=u32 750) -> ()  [unwired: 1 out]
                          n1671 = Array To Cluster(array=w5757) -> (cluster=w5756:T15)
                          n1672 = Bundle By Name(cluster=w5756, "Axes[1]"=1.0) -> (w5759:T15)
                          n1673 = Cluster To Array(cluster=w5759) -> (array=w5758:dbl[])
                          n1674 = global write "Robot Global Data.vi" "Axes"(w5758) -> ()
                        }
                        frame #3 {
                          n1675 = global write "Robot Global Data.vi" "Current State"(FALSE ("Current State")) -> ()
                          n1676 = Wait (ms)(milliseconds to wait=u32 500) -> ()  [unwired: 1 out]
                        }
                      }
                    }
                    frame "L" {
                      n1677 = flat-sequence {
                        tunnel: w5793 -> [w5803]
                        tunnel: w5792 -> [w5808]
                        tunnel: w5791 -> [w5802]
                        tunnel: w5790 -> [w5801]
                        tunnel: [w5807] -> w5789
                        tunnel: [w5806] -> w5788
                        tunnel: [w5805] -> w5786
                        tunnel: [w5804] -> w5784
                        tunnel: w5789 -> [w5817]
                        tunnel: w5788 -> [w5816]
                        tunnel: [w5815] -> w5787
                        tunnel: w5786 -> [w5815]
                        tunnel: [w5814] -> w5785
                        tunnel: w5784 -> [w5814]
                        tunnel: [w5813] -> w5782
                        tunnel: [w5812] -> w5780
                        tunnel: w5787 -> [w5824]
                        tunnel: w5785 -> [w5823]
                        tunnel: [w5822] -> w5783
                        tunnel: w5782 -> [w5822]
                        tunnel: [w5821] -> w5781
                        tunnel: w5780 -> [w5821]
                        tunnel: [w5820] -> w5779
                        tunnel: [w5819] -> w5778
                        tunnel: w5783 -> [w5834]
                        tunnel: w5781 -> [w5833]
                        tunnel: w5779 -> [w5832]
                        tunnel: w5778 -> [w5831]
                        tunnel: [w5830] -> w5777
                        tunnel: [w5829] -> w5776
                        tunnel: [w5827] -> w5775
                        tunnel: [w5826] -> w5774
                        tunnel: [w5840] -> w5773
                        tunnel: [w5839] -> w5772
                        tunnel: [w5838] -> w5771
                        tunnel: [w5837] -> w5770
                        tunnel: w5774 -> [w5837]
                        tunnel: w5775 -> [w5838]
                        tunnel: w5776 -> [w5839]
                        tunnel: w5777 -> [w5840]
                        tunnel: [w5850] -> w5763
                        tunnel: w5773 -> [w5850]
                        tunnel: [w5849] -> w5765
                        tunnel: w5772 -> [w5849]
                        tunnel: [w5848] -> w5767
                        tunnel: w5771 -> [w5848]
                        tunnel: [w5847] -> w5769
                        tunnel: w5770 -> [w5847]
                        tunnel: w5769 -> [w5862]
                        tunnel: [w5862] -> w5768
                        tunnel: w5767 -> [w5861]
                        tunnel: [w5861] -> w5766
                        tunnel: w5765 -> [w5860]
                        tunnel: [w5860] -> w5764
                        tunnel: w5763 -> [w5859]
                        tunnel: [w5859] -> w5762
                        tunnel: w5768 -> [w5863]
                        tunnel: w5766 -> [w5864]
                        tunnel: w5764 -> [w5865]
                        tunnel: w5762 -> [w5866]
                        frame #0 {
                          n1678 = global read "Robot Global Data.vi" "Axes"() -> (w5798:dbl[])
                          n1679 = global write "Robot Global Data.vi" "Lift_Position"(2.0) -> ()
                          n1680 = Wait (ms)(milliseconds to wait=u32 250) -> ()  [unwired: 1 out]
                          n1681 = Array To Cluster(array=w5798) -> (cluster=w5797:T15)
                          n1682 = Bundle By Name(cluster=w5797, "Axes[1]"=-1.0) -> (w5800:T15)
                          n1683 = Cluster To Array(cluster=w5800) -> (array=w5799:dbl[])
                          n1684 = global write "Robot Global Data.vi" "Axes"(w5799) -> ()
                        }
                        frame #1 {
                          n1685 = call "PID Distance.vi"("Distance"=-10.0, "Angle"=-150.0, "RightEncoder"=w5808, "LeftEncoder"=w5801, "GyroDevRef"=w5802, "RobotDriveDevRef"=w5803) -> ("RightEncoder 2"=w5804:T11, "LeftEncoder 2"=w5805:T11, "GyroDevRef 2"=w5806:T8, "RobotDriveDevRef 2"=w5807:T1)  [unwired: 2 in]
                        }
                        frame #2 {
                          n1686 = global write "Robot Global Data.vi" "Lift_Position"(3.0) -> ()
                          n1687 = call "PID turning.vi"("Angle"=-90.0, "GyroDevRef"=w5816, "RobotDriveDevRef"=w5817) -> ("GyroDevRef 2"=w5812:T8, "RobotDriveDevRef 2"=w5813:T1)  [unwired: 7 in]
                        }
                        frame #3 {
                          n1688 = call <vilib>:"WPI_EncoderReset.vi"("EncoderDevRef"=w5824) -> ("EncoderDevRef"=w5820:T11)  [unwired: 9 in, 1 out]
                          n1689 = Wait (ms)(milliseconds to wait=u32 10) -> ()  [unwired: 1 out]
                          n1690 = call <vilib>:"WPI_EncoderReset.vi"("EncoderDevRef"=w5823) -> ("EncoderDevRef"=w5819:T11)  [unwired: 9 in, 1 out]
                        }
                        frame #4 {
                          n1691 = global write "Robot Global Data.vi" "Lift_Position"(3.0) -> ()
                          n1692 = call "PID Distance.vi"("Distance"=30.0, "Angle"=-90.0, "RightEncoder"=w5831, "LeftEncoder"=w5832, "GyroDevRef"=w5833, "RobotDriveDevRef"=w5834) -> ("RightEncoder 2"=w5826:T11, "LeftEncoder 2"=w5827:T11, "GyroDevRef 2"=w5829:T8, "RobotDriveDevRef 2"=w5830:T1)  [unwired: 2 in]
                        }
                        frame #5 {
                          n1693 = global read "Robot Global Data.vi" "Axes"() -> (w5844:dbl[])
                          n1694 = Wait (ms)(milliseconds to wait=u32 500) -> ()  [unwired: 1 out]
                          n1695 = Array To Cluster(array=w5844) -> (cluster=w5843:T15)
                          n1696 = Bundle By Name(cluster=w5843, "Axes[1]"=0.3) -> (w5846:T15)
                          n1697 = Cluster To Array(cluster=w5846) -> (array=w5845:dbl[])
                          n1698 = global write "Robot Global Data.vi" "Axes"(w5845) -> ()
                        }
                        frame #6 {
                          n1699 = global write "Robot Global Data.vi" "Current State"(FALSE ("Current State")) -> ()
                          n1700 = Wait (ms)(milliseconds to wait=u32 400) -> ()  [unwired: 1 out]
                        }
                        frame #7 {
                          n1701 = global read "Robot Global Data.vi" "Axes"() -> (w5856:dbl[])
                          n1702 = Wait (ms)(milliseconds to wait=u32 250) -> ()  [unwired: 1 out]
                          n1703 = Array To Cluster(array=w5856) -> (cluster=w5855:T15)
                          n1704 = Bundle By Name(cluster=w5855, "Axes[1]"=-1.0) -> (w5858:T15)
                          n1705 = Cluster To Array(cluster=w5858) -> (array=w5857:dbl[])
                          n1706 = global write "Robot Global Data.vi" "Axes"(w5857) -> ()
                        }
                        frame #8 {
                          n1707 = call "PID Distance.vi"("Distance"=0.0, "Angle"=-90.0, "RightEncoder"=w5863, "LeftEncoder"=w5864, "GyroDevRef"=w5865, "RobotDriveDevRef"=w5866) -> ()  [unwired: 2 in, 4 out]
                        }
                        frame #9 {
                          n1708 = global write "Robot Global Data.vi" "Lift_Position"(1.0) -> ()
                        }
                      }
                    }
                    frame Default {
                    }
                  }
                }
              }
            }
            frame Default {
              n1709 = flat-sequence {
                tunnel: w5871 -> [w5879]
                tunnel: w5870 -> [w5878]
                tunnel: w5872 -> [w5876]
                tunnel: [w5877] -> w5874
                tunnel: w5873 -> [w5875]
                tunnel: w5874 -> [w5882]
                frame #0 {
                  n1710 = call "PID Distance.vi"("Distance"=90.0, "Angle"=0.0, "RightEncoder"=w5875, "LeftEncoder"=w5876, "GyroDevRef"=w5878, "RobotDriveDevRef"=w5879) -> ("RobotDriveDevRef 2"=w5877:T1)  [unwired: 2 in, 3 out]
                }
                frame #1 {
                  w5883 = 0.0
                  n1711 = call <vilib>:"WPI_RobotDriveTankDrive.vi"("Right axis value"=w5883, "Left axis value"=w5883, "RobotDriveDevRef"=w5882) -> ()  [unwired: 6 in, 3 out]
                }
              }
            }
          }
        }
      }
    }
    frame "Right Scale V" {
      n1712 = flat-sequence {
        tunnel: w5887 -> [w5919]
        tunnel: w5885 -> [w5917]
        tunnel: w5886 -> [w5916]
        tunnel: [w5915] -> w5894
        tunnel: [w5914] -> w5893
        tunnel: [w5913] -> w5892
        tunnel: [w5912] -> w5891
        tunnel: w5888 -> [w5905]
        tunnel: w5884 -> [w5895]
        tunnel: w5889 -> [w5921]
        tunnel: w5894 -> [w5925]
        tunnel: w5893 -> [w5924]
        tunnel: w5892 -> [w5923]
        tunnel: w5891 -> [w5922]
        tunnel: w5890 -> [w5920]
        frame #0 {
          w5918 = 0.0 ("Left axis value")
          n1713 = global read "Robot Global Data.vi" "Axes"() -> (w5898:dbl[])
          n1714 = Multiply(x=w5905, y=1000.0) -> (x*y=w5906:dbl)
          n1715 = global write "Robot Global Data.vi" "Lift_Position"(0.0) -> ()
          n1716 = global write "Robot Global Data.vi" "Current State"(TRUE ("Current State")) -> ()
          n1717 = global write "Robot Global Data.vi" "Raise_Mast"(FALSE ("Current State")) -> ()
          n1718 = Wait (ms)(milliseconds to wait=u32 100) -> ()  [unwired: 1 out]
          n1719 = Array To Cluster(array=w5898) -> (cluster=w5897:T15)
          n1720 = Bundle By Name(cluster=w5897, "Axes[1]"=-1.0) -> (w5900:T15)
          n1721 = Greater?(x=w5906, y=11000.0) -> (0:w5908:bool)
          n1722 = Equal?(x=w5906, y=0.0) -> (x = y?=w5909:bool)
          n1723 = Or(x=w5908, y=w5909) -> ()  [unwired: 1 out]
          n1724 = Cluster To Array(cluster=w5900) -> (array=w5899:dbl[])
          n1725 = call <vilib>:"WPI_GyroReset.vi"("GyroDevRef"=w5916) -> ("GyroDevRef"=w5912:T8)  [unwired: 9 in, 1 out]
          n1726 = call <vilib>:"WPI_EncoderReset.vi"("EncoderDevRef"=w5895) -> ("EncoderDevRef"=w5914:T11)  [unwired: 9 in, 1 out]
          n1727 = global write "Robot Global Data.vi" "Axes"(w5899) -> ()
          n1728 = call <vilib>:"WPI_EncoderReset.vi"("EncoderDevRef"=w5917) -> ("EncoderDevRef"=w5913:T11)  [unwired: 9 in, 1 out]
          n1729 = call <vilib>:"WPI_RobotDriveTankDrive.vi"("Right axis value"=w5918, "Left axis value"=w5918, "RobotDriveDevRef"=w5919) -> ("RobotDriveDevRef"=w5915:T1)  [unwired: 6 in, 2 out]
        }
        frame #1 {
          n1730 = case shown="\"L\"" w5921 {
            tunnel: w5925 -> [w5935 w6309 w6644]
            tunnel: w5924 -> [w5938 w6306 w6646]
            tunnel: w5923 -> [w5937 w6307 w6645]
            tunnel: w5922 -> [w5936 w6308 w6643]
            tunnel: w5920 -> [w5934 w6305 _]
            frame "L" {
              n1731 = flat-sequence {
                tunnel: [w5990] -> w5982
                tunnel: [w5989] -> w5981
                tunnel: [w5987] -> w5980
                tunnel: [w5988] -> w5979
                tunnel: w5938 -> [w5983]
                tunnel: w5937 -> [w5984]
                tunnel: w5936 -> [w5985]
                tunnel: w5935 -> [w5986]
                tunnel: w5982 -> [w6001]
                tunnel: w5981 -> [w6002]
                tunnel: [w6005] -> w5978
                tunnel: w5980 -> [w6005]
                tunnel: [w6004] -> w5977
                tunnel: w5979 -> [w6004]
                tunnel: [w5999] -> w5976
                tunnel: [w6000] -> w5975
                tunnel: w5978 -> [w6012]
                tunnel: w5977 -> [w6011]
                tunnel: [w6010] -> w5974
                tunnel: [w6009] -> w5973
                tunnel: [w6008] -> w5972
                tunnel: w5976 -> [w6008]
                tunnel: [w6006] -> w5971
                tunnel: w5975 -> [w6006]
                tunnel: w5974 -> [w6017]
                tunnel: w5973 -> [w6018]
                tunnel: w5972 -> [w6019]
                tunnel: [w6015] -> w5970
                tunnel: [w6016] -> w5969
                tunnel: w5971 -> [w6020]
                tunnel: [w6013] -> w5968
                tunnel: [w6014] -> w5967
                tunnel: w5970 -> [w6032]
                tunnel: w5969 -> [w6031]
                tunnel: [w6030] -> w5966
                tunnel: [w6029] -> w5965
                tunnel: [w6035] -> w5964
                tunnel: w5968 -> [w6035]
                tunnel: [w6034] -> w5963
                tunnel: w5967 -> [w6034]
                tunnel: w5966 -> [w6041]
                tunnel: [w6041] -> w5962
                tunnel: [w6040] -> w5961
                tunnel: [w6039] -> w5960
                tunnel: [w6038] -> w5959
                tunnel: w5965 -> [w6038]
                tunnel: w5964 -> [w6037]
                tunnel: w5963 -> [w6036]
                tunnel: w5962 -> [w6049]
                tunnel: [w6046] -> w5958
                tunnel: w5961 -> [w6048]
                tunnel: w5960 -> [w6047]
                tunnel: w5959 -> [w6050]
                tunnel: [w6045] -> w5957
                tunnel: [w6044] -> w5956
                tunnel: [w6043] -> w5955
                tunnel: w5958 -> [w6057]
                tunnel: [w6056] -> w5933
                tunnel: w5957 -> [w6054]
                tunnel: [w6053] -> w5931
                tunnel: w5956 -> [w6059]
                tunnel: [w6059] -> w5929
                tunnel: w5955 -> [w6058]
                tunnel: [w6058] -> w5927
                tunnel: w5933 -> [w6065]
                tunnel: [w6065] -> w5932
                tunnel: w5931 -> [w6064]
                tunnel: [w6064] -> w5930
                tunnel: w5929 -> [w6063]
                tunnel: [w6061] -> w5928
                tunnel: w5927 -> [w6062]
                tunnel: [w6060] -> w5926
                tunnel: w5932 -> [w6076]
                tunnel: [w6070] -> w5954
                tunnel: [w6069] -> w5953
                tunnel: w5930 -> [w6069]
                tunnel: [w6068] -> w5952
                tunnel: w5928 -> [w6068]
                tunnel: [w6067] -> w5951
                tunnel: w5926 -> [w6067]
                tunnel: w5954 -> [w6083]
                tunnel: [w6083] -> w5950
                tunnel: w5953 -> [w6082]
                tunnel: [w6082] -> w5949
                tunnel: w5952 -> [w6081]
                tunnel: [w6081] -> w5948
                tunnel: w5951 -> [w6080]
                tunnel: [w6080] -> w5947
                tunnel: [w6089] -> w5946
                tunnel: [w6088] -> w5945
                tunnel: [w6087] -> w5944
                tunnel: [w6086] -> w5943
                tunnel: w5947 -> [w6095]
                tunnel: w5948 -> [w6096]
                tunnel: w5949 -> [w6084]
                tunnel: w5950 -> [w6085]
                tunnel: w5946 -> [w6103]
                tunnel: [w6103] -> w5942
                tunnel: w5945 -> [w6102]
                tunnel: [w6102] -> w5941
                tunnel: w5944 -> [w6101]
                tunnel: [w6101] -> w5940
                tunnel: w5943 -> [w6100]
                tunnel: [w6100] -> w5939
                tunnel: w5942 -> [w6108]
                tunnel: w5941 -> [w6107]
                tunnel: w5940 -> [w6105]
                tunnel: w5939 -> [w6106]
                tunnel: w5934 -> [w6104]
                frame #0 {
                  n1732 = while {
                    stop <- w5993 stop-if-true
                    w5994 = 20.0 ("y")
                    n1733 = global read "Robot Global Data.vi" "Distance 2"() -> (w5995:dbl)
                    n1734 = global read "Robot Global Data.vi" "Distance"() -> (w5996:dbl)
                    n1735 = Greater?(x=w5996, y=w5994) -> (0:w5998:bool)
                    n1736 = Greater?(x=w5995, y=w5994) -> (0:w5997:bool)
                    n1737 = And(x=w5998, y=w5997) -> (x .and. y?=w5993:bool)
                    n1738 = global write "Robot Global Data.vi" "Raise_Mast"(w5993) -> ()
                  }
